vi "read tag by index.vi"(8 "error in":errorcluster, 10 "index":i32, 11 "tag collection in":refnum<class "tag collection.lvclass">) -> (0 "error out":errorcluster, 1 "tag":refnum<class "tag descriptor.lvclass">, 3 "tag collection out":refnum<class "tag collection.lvclass">)   [LabVIEW 2013, in "tag bus.lvlib" / "tag collection.lvclass"]
uses:
  tag collection.lvclass
  tag/tag descriptor.lvclass
  tag collection.lvclass/tag collection.ctl
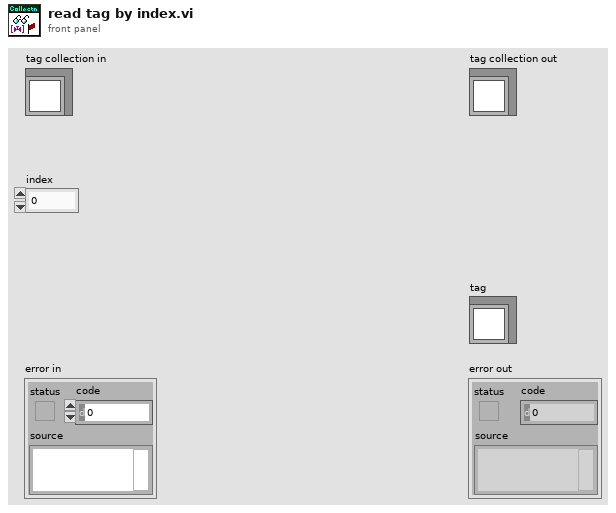
[diagram p1: front panel]
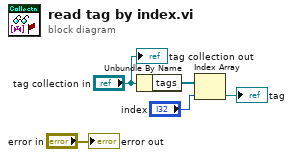
[diagram p0: block diagram]
diagram:
  n1 = Unbundle By Name("tag collection in") -> ("tags"=w3:refnum<class "tag descriptor.lvclass">[])
  n2 = Index Array(array=w3, index="index") -> (element=→"tag":refnum<class "tag descriptor.lvclass">)
  "error out" <- "error in"
  "tag collection out" <- "tag collection in"
